vi "Arterial pressure to HR - Copy.vi"(9 "Sampling Rate":dbl, 11 "Raw HR":dbl[](array[numeric])) -> (3 "HR":dbl[](array[numeric]))   [LabVIEW 2014]
uses:
  <vilib>/Analysis/baseanly.llb/Mean (DBL).vi
  <vilib>/addons/System Identification/Data Preprocess.llb/SI Bandpass Filter (SISO Array).vi
  <vilib>/addons/System Identification/NI_SysID.lvlib
  <vilib>/Analysis/NI_AAL_SigProc.lvlib
  <vilib>/Analysis/NI_AALBase.lvlib
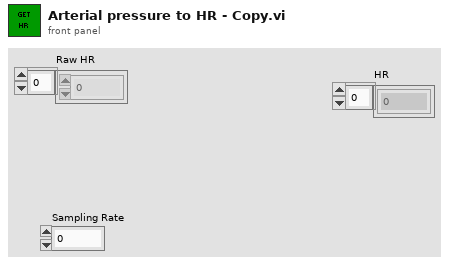
[diagram p1: front panel]
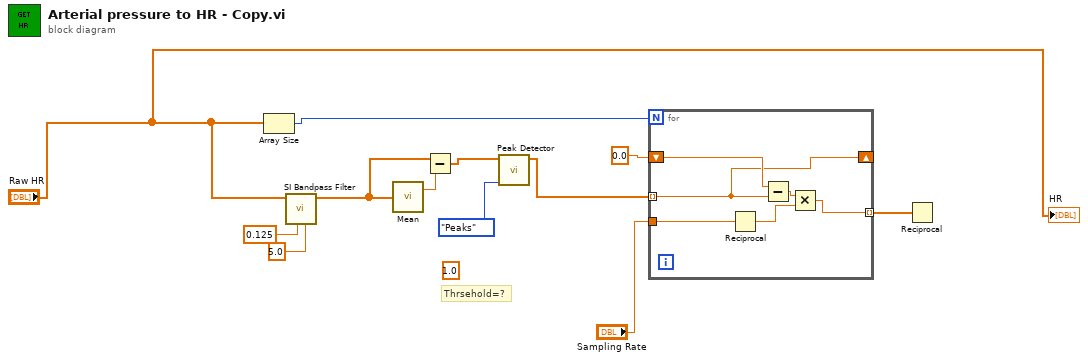
[diagram p0: block diagram]
diagram:
  (unwired) 1.0 ("threshold")
  # "Thrsehold=?"
  n1 = Array Size(array="Raw HR") -> (size(s)=w2:i32)
  n2 = call-poly <vilib>:"SI Bandpass Filter.vi"("high cutoff freq"=5.0, "low cutoff freq"=0.125, "stimulus signal in"="Raw HR") -> ("stimulus signal out"=w10:dbl[])  [unwired: 6 in, 2 out]
  n3 = call-poly <vilib>:"Mean.vi"("X"=w10) -> ("mean"=w9:dbl)  [unwired: 1 out]
  n4 = Subtract(x=w10, y=w9) -> (x-y=w8:dbl[])
  n5 = call <vilib>:"Peak Detector.vi"("peaks/valleys"=enum32{"Peaks", "Valleys"}."Peaks", "X"=w8) -> ("Locations"=w5:dbl[])  [unwired: 5 in, 4 out]
  n6 = for {
    N: w2 -> [_]
    shift-right: [w15] -> _
    shift-left: 0.0 -> [w16]
    tunnel: w5 -> [w15] mode=indexing
    tunnel: "Sampling Rate" -> [w14]
    tunnel: [w13] -> w3 mode=indexing
    n7 = Reciprocal(x=w14) -> (1/x=w17:dbl)
    n8 = Subtract(x=w16, y=w15) -> (x-y=w18:dbl)
    n9 = Multiply(x=w18, y=w17) -> (x*y=w13:dbl)
  }
  n10 = Reciprocal(x=w3) -> ()  [unwired: 1 out]
  "HR" <- "Raw HR"
